vi "Close.vi"(8 "error in (no error)":errorcluster, 11 "EventHandler in":refnum<class "EventHandler.lvclass">) -> (0 "error out":errorcluster, 3 "EventHandler out":refnum<class "EventHandler.lvclass">)   [LabVIEW 2020, in "Volatus.lvlib" / "EventHandler.lvclass"]
uses:
  EventHandler.lvclass
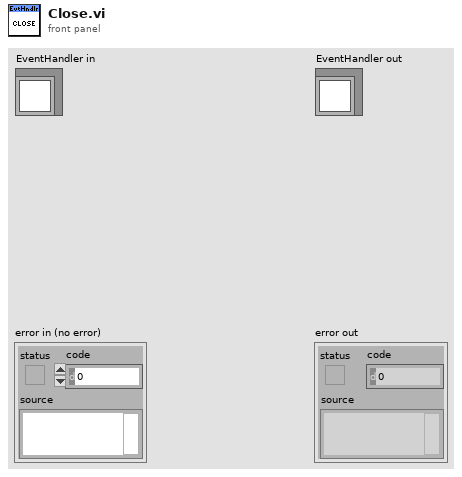
[diagram p1: front panel]
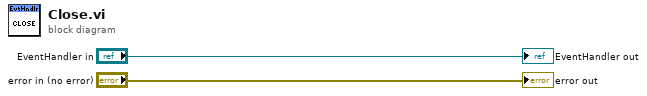
[diagram p0: block diagram]
diagram:
  "error out" <- "error in (no error)"
  "EventHandler out" <- "EventHandler in"
